vi "Start Game.vi"(8 "error in (no error)":errorcluster, 11 "Game in":refnum<class "Game.lvclass">) -> (0 "error out":errorcluster, 3 "Game out":refnum<class "Game.lvclass">)   [LabVIEW 2020, in "SquareBattle.lvlib" / "Game.lvclass"]
uses:
  Game.lvclass
  Game.lvclass/Game.ctl
  Team/Team.lvclass
  Map/Map.lvclass
  Square/Square.lvclass
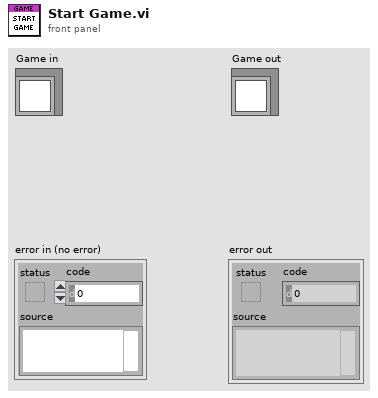
[diagram p1: front panel]
types:
  T1 = typedef "SquareBattle.lvlib/Position.ctl" = cluster{"Row":i32, "Col":i32}
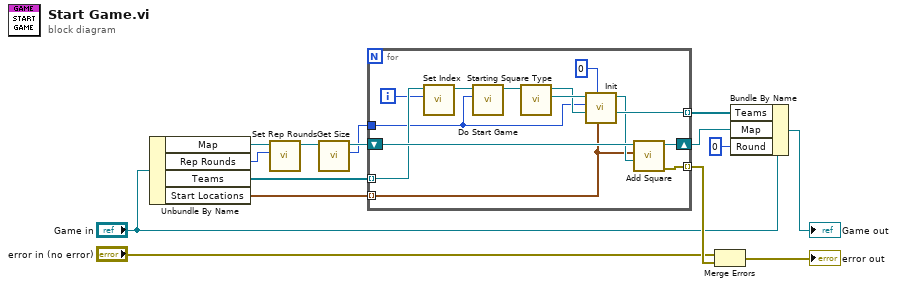
[diagram p0: block diagram]
diagram:
  n1 = Unbundle By Name("Game in") -> ("Map"=w3:refnum<class "Map.lvclass">, "Rep Rounds"=w1:u32, "Teams"=w7:refnum<class "Team.lvclass">[], "Start Locations"=w6:T1[])
  n2 = call "Set Rep Rounds.vi"("Rep Rounds"=w1, "Map in"=w3) -> ("Map out"=w2:refnum<class "Map.lvclass">)  [unwired: 8 in, 1 out]
  n3 = call "Get Size.vi"("Map in"=w2) -> ("Size"=w4:i32, "Map out"=w5:refnum<class "Map.lvclass">)  [unwired: 9 in]
  n4 = for {
    shift-right: [w28] -> w13
    shift-left: w5 -> [w29]
    tunnel: w4 -> [w16]
    tunnel: [w25] -> w11 mode=indexing
    tunnel: [w27] -> w15 mode=indexing
    tunnel: w7 -> [w23] mode=indexing
    tunnel: w6 -> [w19] mode=indexing
    i -> [w22]
    n5 = call "Set Index.vi"("Index"=w22, "Team in"=w23) -> ("Team out"=w18:refnum<class "Team.lvclass">)  [unwired: 9 in]
    n6 = call "Do Start Game.vi"("Board Size"=w16, "Team in"=w18) -> ("Team out"=w17:refnum<class "Team.lvclass">)  [unwired: 9 in]
    n7 = call-dynamic "Starting Square Type.vi"("Team in"=w17) -> ("Square"=w21:refnum<class "Square.lvclass">, "Team out"=w20:refnum<class "Team.lvclass">)  [unwired: 9 in]
    n8 = call "Init.vi"("Position"=w19, "Round"=u32 0, "Team in"=w20, "Board Size"=w16, "Square in"=w21) -> ("Team out"=w25:refnum<class "Team.lvclass">, "Square out"=w24:refnum<class "Square.lvclass">)  [unwired: 5 in]
    n9 = call "Add Square.vi"("Square"=w24, "Position"=w19, "Map in"=w29) -> ("error out"=w27:errorcluster, "Map out"=w28:refnum<class "Map.lvclass">)  [unwired: 7 in]
  }
  n10 = Merge Errors("error in (no error)", w15) -> (→"error out":errorcluster)
  n11 = Bundle By Name(cluster="Game in", "Teams"=w11, "Map"=w13, "Round"=u32 0) -> (→"Game out":refnum<class "Game.lvclass">)
